vi "Top Level FPGA_w8randLED.vi"() -> ()   [LabVIEW 2012]
uses:
  <vilib>/Platform/TimedLoop/XDataNode/timing_clust.ctl
  <vilib>/Platform/TimedLoop/XDataNode/nitl_modes.ctl
  <vilib>/Platform/TimedLoop/XDataNode/wakeup.ctl
  <vilib>/rvi/DataTransferAndStorage/Container/Common/niFpgaContainerMetaDataKey.ctl
  <vilib>/rvi/DataTransferAndStorage/Container/Common/niFpgaContainerState.ctl
  <vilib>/rvi/DataTransferAndStorage/Container/Common/niFpgaDataTypeControl.ctl
  <vilib>/rvi/DataTransferAndStorage/Container/Common/niFpgaContainerImplementationControl.ctl
  <vilib>/rvi/DataTransferAndStorage/Container/Common/niFpgaContainerArbitrationOptionsControl.ctl
  <vilib>/rvi/DataTransferAndStorage/Container/Common/niFpgaTransferTypeControl.ctl
  <vilib>/rvi/DataTransferAndStorage/Container/Common/niFpgaContainerInitializationParameters.ctl
  <vilib>/rvi/Memory/Memory_Types/niFpgaMemoryInterfaceConfiguration.ctl
  <vilib>/rvi/FIFO/Fifo_Types/niFpgaFifoControlLogicControl.ctl
  <vilib>/rvi/eio/common/nirviEmuTemplateMethod_errors.vi
  <vilib>/rvi/FIFO/Fifo_Resource/nirvififoEmulationSetSize.vi
  <vilib>/rvi/DataTransferAndStorage/Container/Common/niFpgaContainerGetUniqueNameForEmu.vi
  <vilib>/rvi/Emulation/niFpgaSctlEmulationRegisterWithScheduler.vi
  <vilib>/rvi/DataTransferAndStorage/Container/Common/niFpgaContainerSetEmuInfo.vi
  <vilib>/rvi/eio/common/nirviEmuReportErrorAndStop.vi
  <vilib>/rvi/Emulation/niFpgaSctlEmulationScheduler.vi
  <vilib>/rvi/Emulation/niFpgaSctlEmulationFifoFullMgr.vi
  <vilib>/rvi/errors/niFpgaSetErrorForExecOnDevCompSimple.vi
  <vilib>/rvi/Memory/Memory_Emulation/nirvimemoryEmulationManagerCache_GetValue.vi
  <vilib>/rvi/Memory/Memory_Emulation/niFpgaMemoryEmulationValidateCache.vi
  <vilib>/rvi/Memory/Memory_Emulation/nirvimemoryEmulationManagerCache_InsertValue.vi
  <vilib>/rvi/Memory/Memory_Emulation/nirvimemoryEmulationManagerCache_SetValue.vi
  <vilib>/rvi/Emulation/niFpgaSctlEmulationResourceMgr.vi
  <vilib>/rvi/Memory/Memory_Emulation/niFpgaMemoryEmulationCacheClearOnFirstRun.vi
  <vilib>/rvi/Memory/Memory_Emulation/nirvimemoryEmulationManagerCache_MakeExclusive.vi
  <vilib>/rvi/Memory/Memory_Emulation/nirvimemoryEmulationManagerCache_ReleaseExclusive.vi
  <vilib>/Utility/error.llb/Clear Errors.vi
  <vilib>/eio/EIONode/EIONode.xnode
  <vilib>/rvi/DataTransferAndStorage/Container/XNode/niFpgaContainer.xnode
  <vilib>/rvi/FIFO/Fifo_Resource/nirvififoEmulationClear.vi
  <vilib>/Platform/TimedLoop/XDataNode/XDataNode.xnode
  <vilib>/rvi/LocalResourceManager/LocalResourceManager.xnode
  <vilib>/rvi/FIFO/Fifo_Resource/nirvififoEmulationRead.vi
  <vilib>/rvi/DataTransferAndStorage/Register/Emulation/niFpgaRegisterEmulation.vi
  <vilib>/rvi/Memory/Memory_Emulation/nirvimemoryEmulation.vi
  <vilib>/rvi/FIFO/Fifo_Resource/nirvififoEmulationWrite.vi
  <vilib>/Platform/TimedLoop/XDataNode/XDNodeRunTimeDep.lvlib
panel:
  out "Total number of pulses sent":u64
  in  "location":i16(ring) items=["Purdue", "NIKHEF", "Zurich", "???"]
  in  "Testpulse duration (20 ns ticks)":u32
  in  "initial value":u64
  in  "channel 7 on/off":bool
  in  "channel 6 on/off":bool
  in  "channel 5 on/off":bool
  in  "channel 4 on/off":bool
  in  "channel 3 on/off":bool
  in  "channel 1 on/off":bool
  in  "channel 2 on/off":bool
  in  "channel 0 on/off":bool
  out "Timestamp":u64
  in  "Stop FPGA and exit":bool
  out "DMA FIFO Timed Out?":bool
  in  "Testpulser On/Off":bool
  in  "Testpulse Time Delay (20 ns ticks)":u32=15
  in  "circular buffer length":u32=1000
  in  "# of pretrigger":u32=20
  out "IO Module\\Pll Unlocked":bool
  out "IO Module\\ADC Error B":bool
  out "IO Module\\ADC Error A":bool
  out "Init Done":bool
  in  "Trigger 4":i16=4000
  in  "Trigger 5":i16=4000
  in  "Trigger 6":i16=4000
  in  "Trigger 7":i16=4000
  in  "Trigger 2":i16=4000
  in  "Trigger 3":i16=4000
  in  "Trigger 1":i16=4000
  in  "Record Size only data":u32=95
  in  "Trigger 0":i16=4000
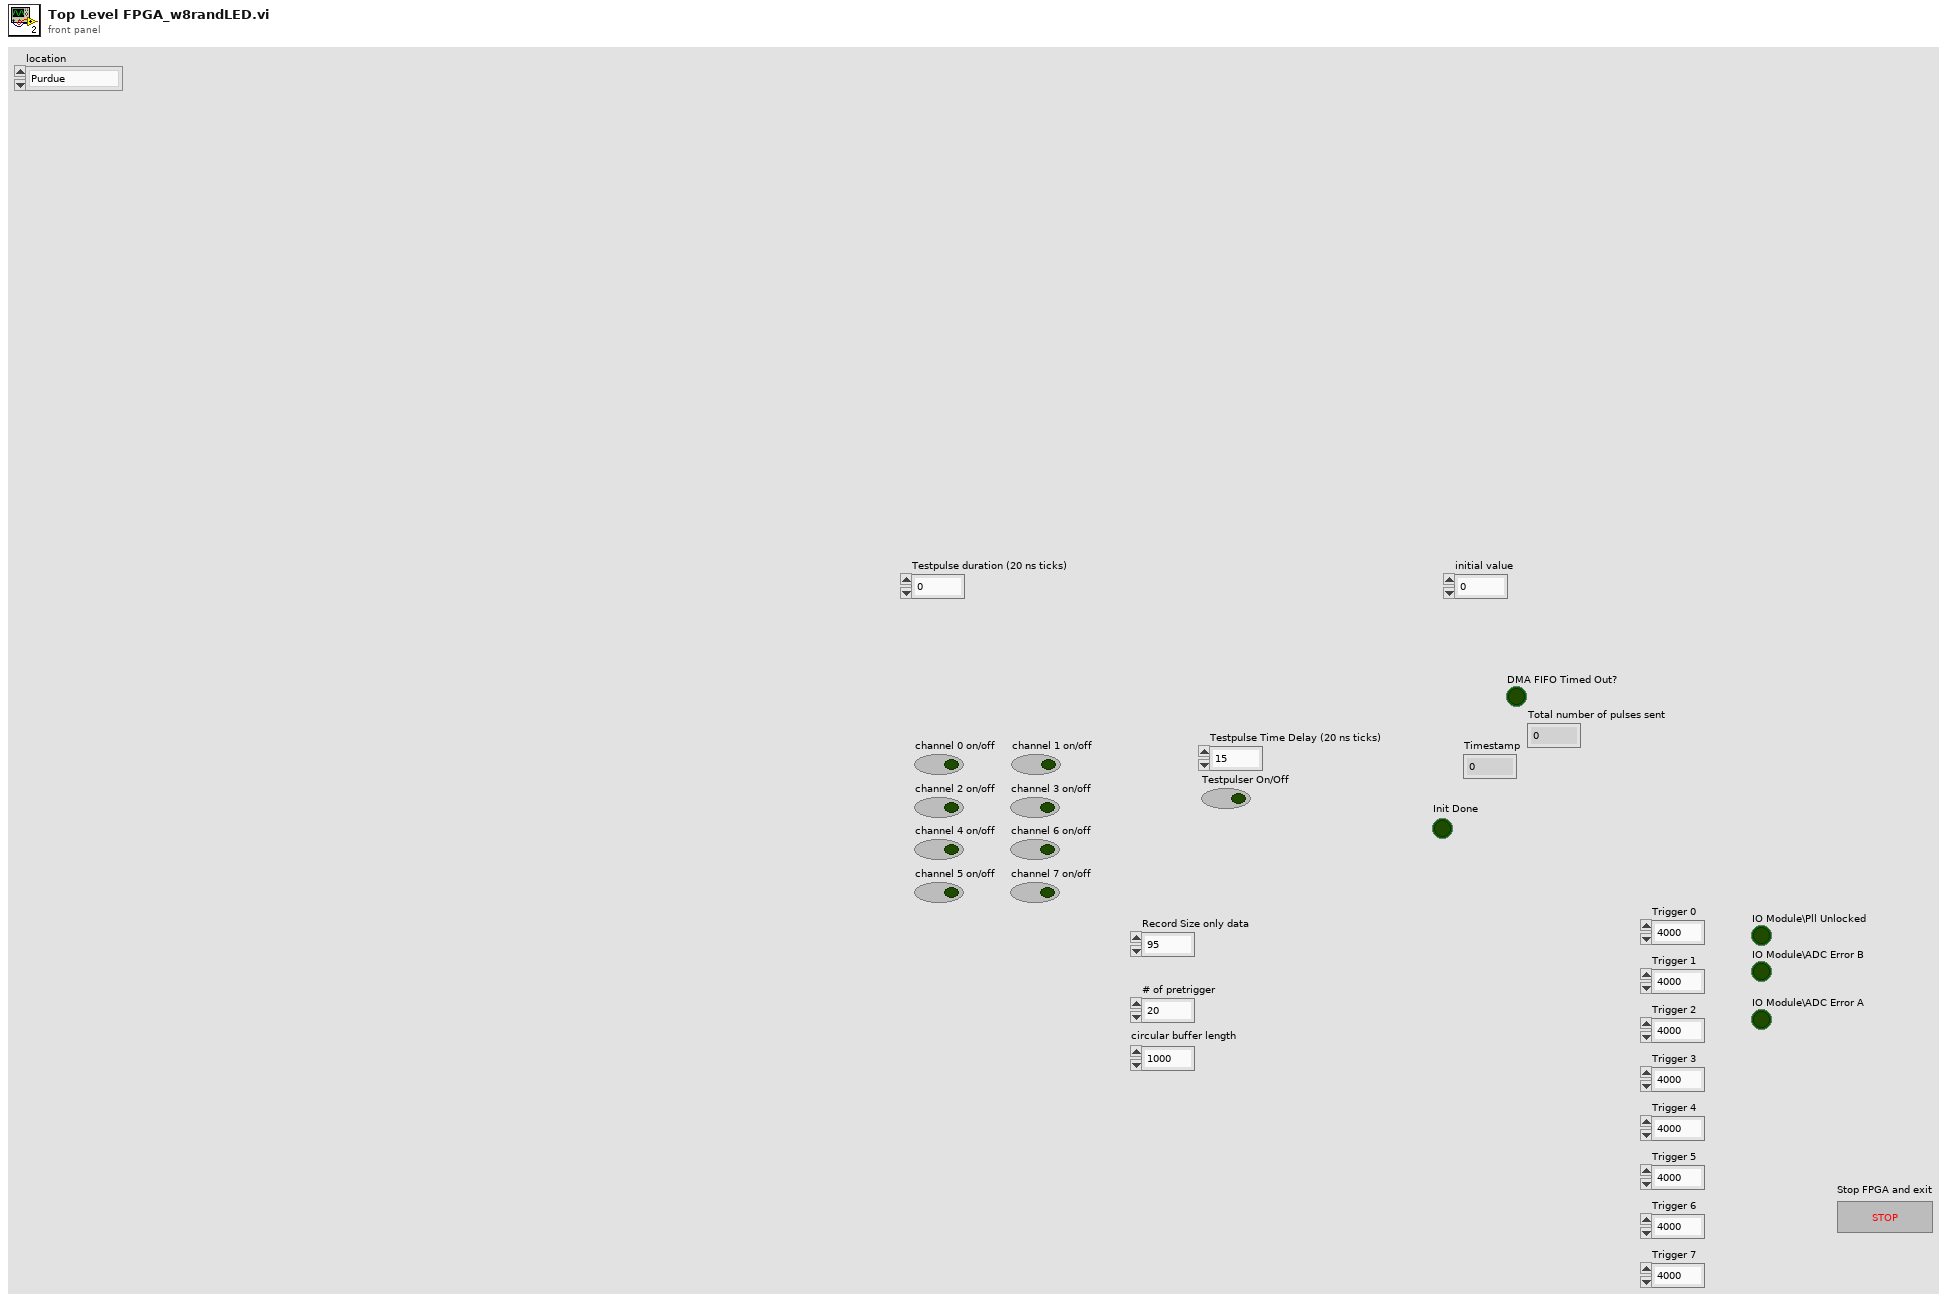
[diagram p1: front panel]
types:
  T1 = typedef "XDNodeRunTimeDep.lvlib/timing_clust.ctl" = cluster{"Expected End [f-1]":u64, "Actual End [f-1]":u64, "Finished Late? [f-1]":bool, "Expected End [i-1]":u64, "Actual End [i-1]":u64, "Finished Late? [i-1]":bool, "Expected Start [i]":u64, "Actual Start [i]":u64, "Expected Start [f]":u64, "Actual Start [f]":u64, "Source Name":string, "Structure Name":string, "Period":i64, "Deadline":i64, "Offset":i64, "Start":i64, "Priority":i32, "Timeout":i32, "Mode":T2, "Wakeup Reason":T3, "Error":errorcluster, "Source Type":string, "Secondary Source Type":string, "Global End Time":u64, "Global Start Time":u64, "Frame Duration":u64, "Iteration Duration":u64, "Assigned CPU":i32, "I/O Scan Engine Mode":u32}
  T2 = typedef "XDNodeRunTimeDep.lvlib/nitl_modes.ctl" = enum32{"No Change", "Process missed periods, maintain original phase", "Discard missed periods, maintain original phase", "Process missed periods, ignore original phase", "Discard missed periods, ignore original phase"}
  T3 = typedef "XDNodeRunTimeDep.lvlib/wakeup.ctl" = enum32{"Normal", "Aborted", "Asynchronous wakeup", "Timing source error", "Timed loop error", "Timeout"}
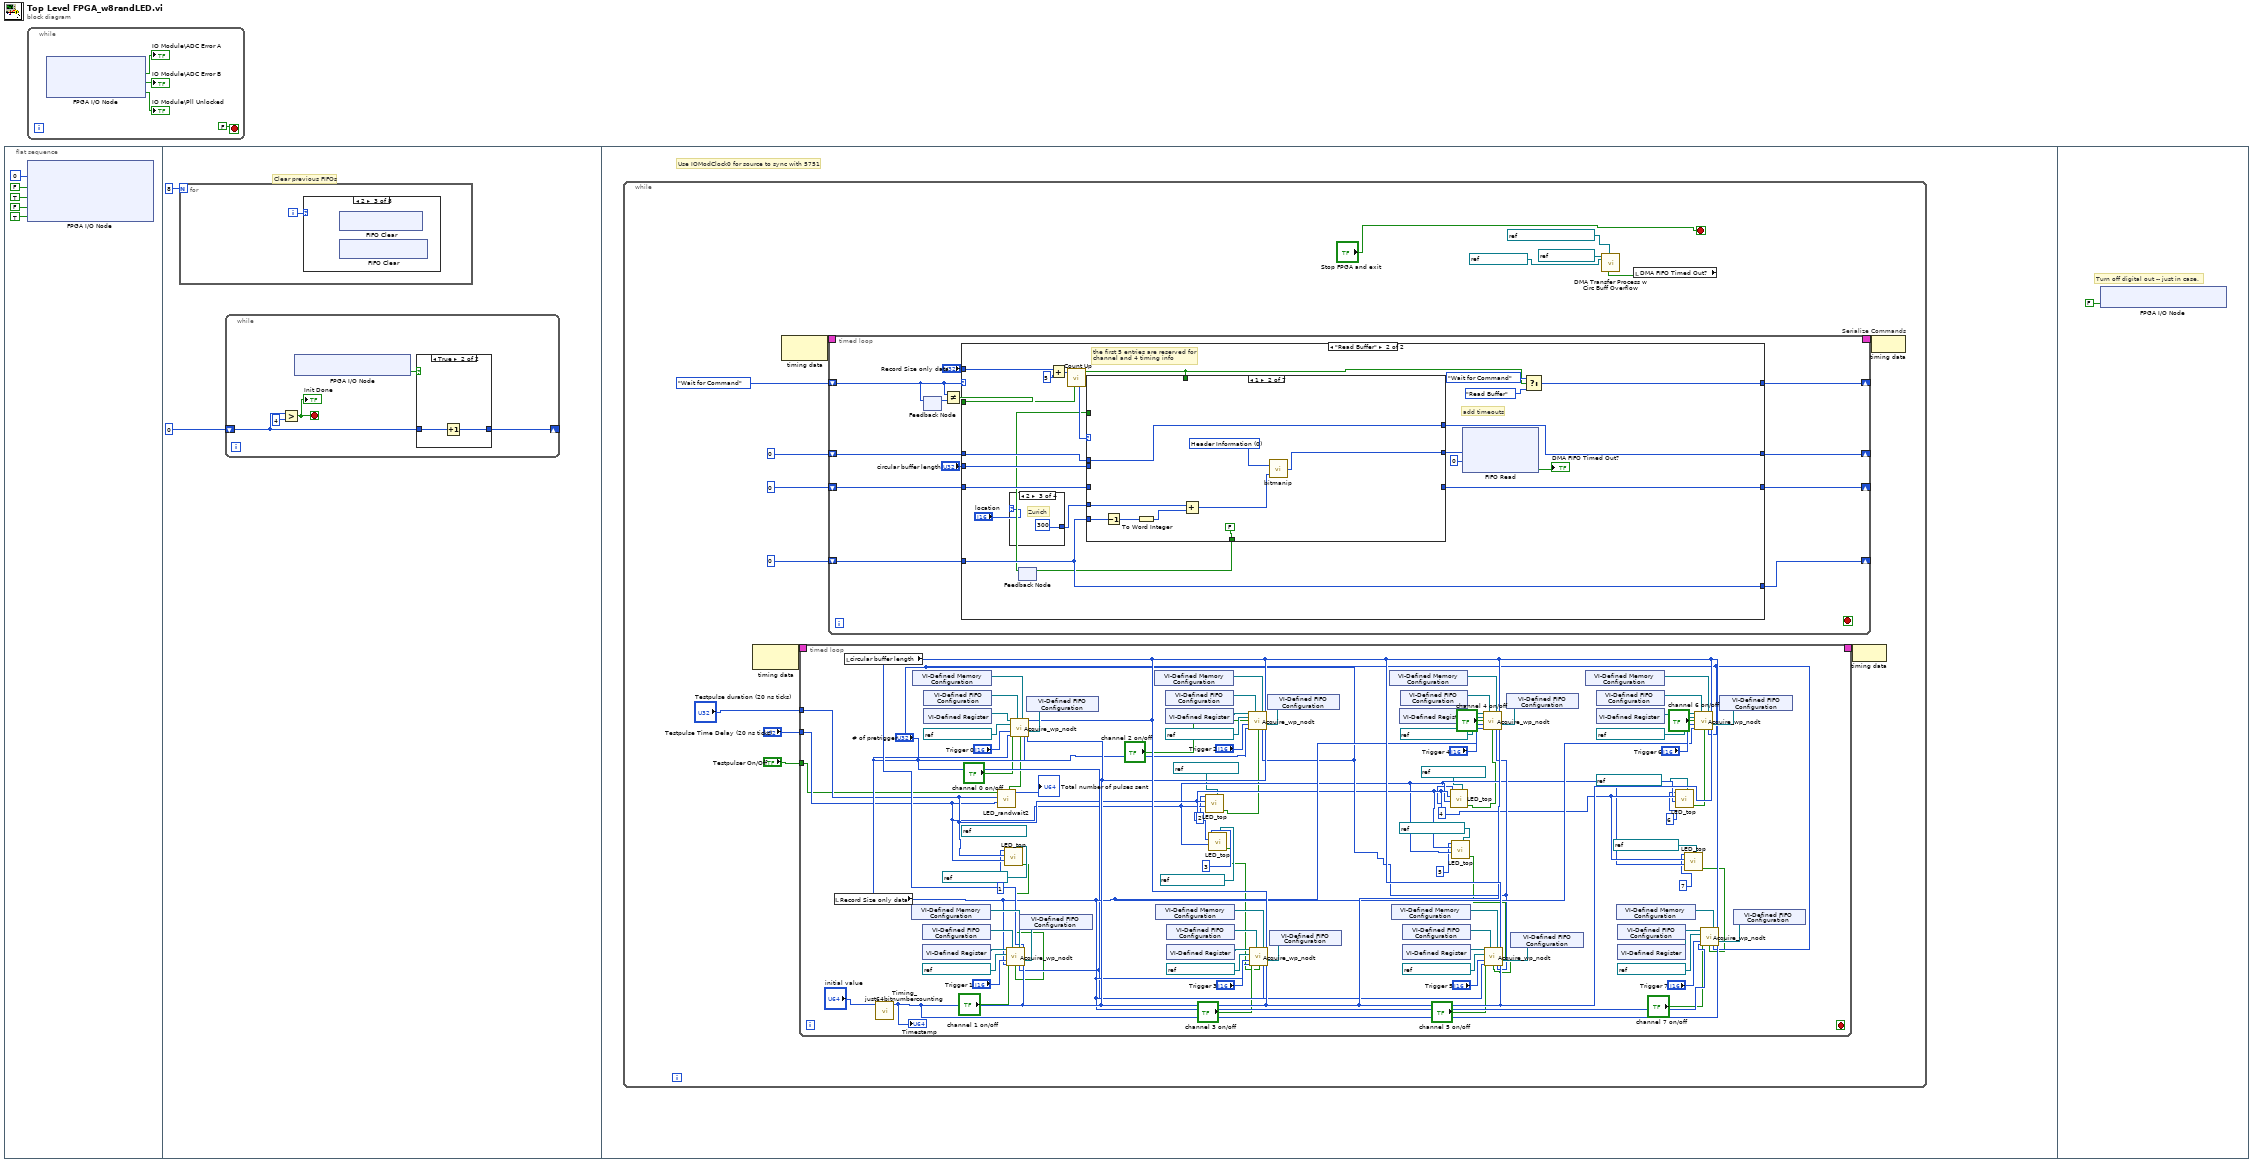
[diagram p0: block diagram]
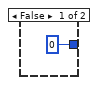
[diagram p2: hidden frame]
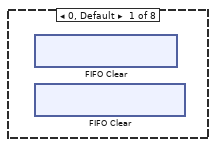
[diagram p3: hidden frame]
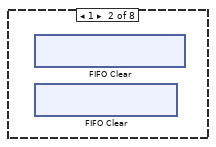
[diagram p4: hidden frame]
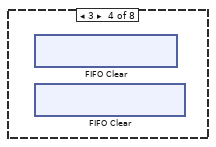
[diagram p5: hidden frame]
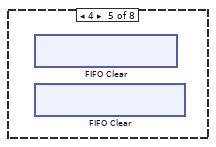
[diagram p6: hidden frame]
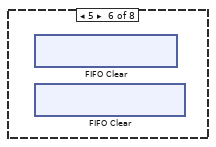
[diagram p7: hidden frame]
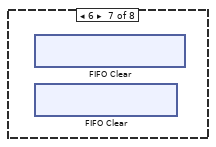
[diagram p8: hidden frame]
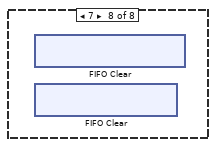
[diagram p9: hidden frame]
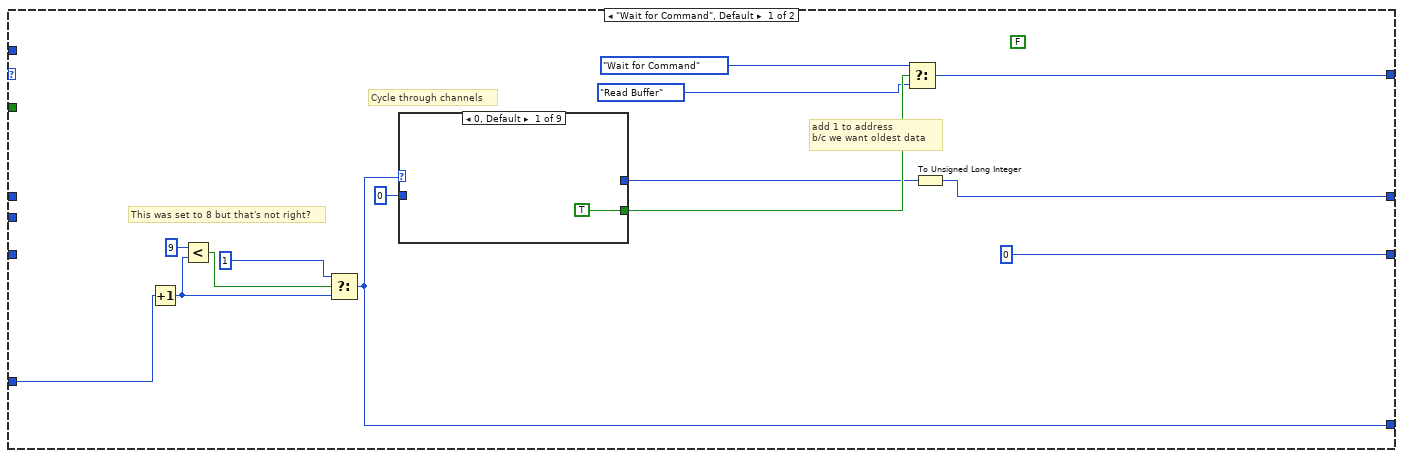
[diagram p10: hidden frame]
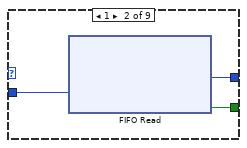
[diagram p11: hidden frame]
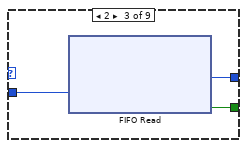
[diagram p12: hidden frame]
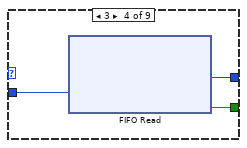
[diagram p13: hidden frame]
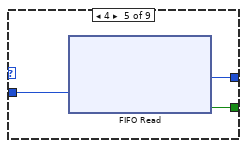
[diagram p14: hidden frame]
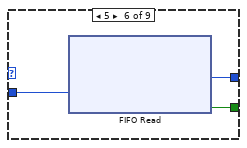
[diagram p15: hidden frame]
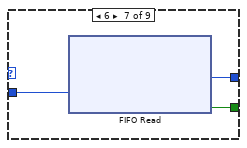
[diagram p16: hidden frame]
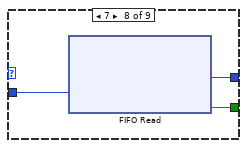
[diagram p17: hidden frame]
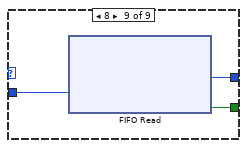
[diagram p18: hidden frame]
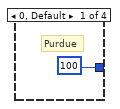
[diagram p19: hidden frame]
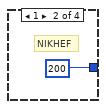
[diagram p20: hidden frame]
diagram:
  n1 = flat-sequence {
    frame #0 {
      n2 = xnode "FPGA I/O Node"("IO Module\\Sample Clock Select"=u8 0 ("IO Module\\Sample Clock Select"), "IO Module\\Force Initialization"=FALSE ("IO Module\\Force Initialization"), "IO Module\\Force Initialization"=TRUE ("IO Module\\Force Initialization"), "IO Module\\Force Initialization"=FALSE ("IO Module\\Force Initialization"), "IO Module\\Digital Output Enable"=TRUE ("IO Module\\Digital Output Enable")) -> ()  [unwired: 5 in, 5 out]
    }
    frame #1 {
      # "Clear previous FIFOs"
      n3 = for {
        N: 8 -> [_]
        i -> [w16]
        n4 = case shown="2" w16 {
          frame 0, Default {
            n5 = xnode ("FIFO Clear")() -> ()  [unwired: 1 in, 1 out]
            n6 = xnode ("FIFO Clear")() -> ()  [unwired: 1 in, 1 out]
          }
          frame 1 {
            n7 = xnode ("FIFO Clear")() -> ()  [unwired: 1 in, 1 out]
            n8 = xnode ("FIFO Clear")() -> ()  [unwired: 1 in, 1 out]
          }
          frame 2 {
            n9 = xnode ("FIFO Clear")() -> ()  [unwired: 1 in, 1 out]
            n10 = xnode ("FIFO Clear")() -> ()  [unwired: 1 in, 1 out]
          }
          frame 3 {
            n11 = xnode ("FIFO Clear")() -> ()  [unwired: 1 in, 1 out]
            n12 = xnode ("FIFO Clear")() -> ()  [unwired: 1 in, 1 out]
          }
          frame 4 {
            n13 = xnode ("FIFO Clear")() -> ()  [unwired: 1 in, 1 out]
            n14 = xnode ("FIFO Clear")() -> ()  [unwired: 1 in, 1 out]
          }
          frame 5 {
            n15 = xnode ("FIFO Clear")() -> ()  [unwired: 1 in, 1 out]
            n16 = xnode ("FIFO Clear")() -> ()  [unwired: 1 in, 1 out]
          }
          frame 6 {
            n17 = xnode ("FIFO Clear")() -> ()  [unwired: 1 in, 1 out]
            n18 = xnode ("FIFO Clear")() -> ()  [unwired: 1 in, 1 out]
          }
          frame 7 {
            n19 = xnode ("FIFO Clear")() -> ()  [unwired: 1 in, 1 out]
            n20 = xnode ("FIFO Clear")() -> ()  [unwired: 1 in, 1 out]
          }
        }
      }
      n21 = while {
        shift-right: [w11] -> _
        shift-left: u16 0 -> [w10]
        stop <- w8 stop-if-true
        n22 = Greater?(x=w10, y=u16 4) -> (0:w8:bool)
        "Init Done" <- w8
        n23 = xnode "FPGA I/O Node"() -> ("IO Module\\Initialization Done"=w12:bool)  [unwired: 1 in, 1 out]
        n24 = case shown="True" w12 {
          tunnel: [u16 0 w15] -> w11
          tunnel: w10 -> [_ w14]
          frame False {
          }
          frame True {
            n25 = Increment(x=w14) -> (x+1=w15:u16)
          }
        }
      }
    }
    frame #2 {
      # "Use IOModClock0 for source to sync with 5751"
      n26 = while {
        stop <- "Stop FPGA and exit" stop-if-true
        n27 = node-c288() -> (w25:T1)  [unwired: 1 in]
        n28 = node-c288() -> (w27:T1)  [unwired: 1 in]
        n29 = timed-loop {
          timing: w25 -> [_]
          timing-out: [_] -> w24
          tunnel: "Testpulser On/Off" -> [w35]
          tunnel: "Testpulse Time Delay (20 ns ticks)" -> [w66]
          tunnel: "Testpulse duration (20 ns ticks)" -> [w67]
          stop <- _ stop-if-true
          (unwired) refnum<k21> "IO Module\\D0 0" ("FPGA I/O In")
          n30 = local read "Record Size only data"() -> (w70:u32)
          n31 = local read "circular buffer length"() -> (w72:u32)
          n32 = call "Timing_just64bitnumbercounting.vi"("initial value"="initial value") -> ("x+1"=w71:u64)  [unwired: 10 in]
          "Timestamp" <- w71
          n33 = xnode "VI-Defined Memory Configuration"() -> ("Memory Out"=w118:refnum<k21>)
          n34 = xnode "VI-Defined Memory Configuration"() -> ("Memory Out"=w73:refnum<k21>)
          n35 = xnode "VI-Defined FIFO Configuration"() -> ("FIFO Out"=w117:refnum<k21>)
          n36 = xnode "VI-Defined Register"() -> ("Register Out"=w98:refnum<k21>)
          n37 = xnode "VI-Defined FIFO Configuration"() -> ("FIFO Out"=w74:refnum<k21>)
          n38 = xnode "VI-Defined Register"() -> ("Register Out"=w69:refnum<k21>)
          n39 = call "LED_randwait2.vi"("Testpulse Time Delay (20 ns ticks)"=w66, "Testpulse duration (20 ns ticks)"=w67, "Testpulser On/Off"=w35) -> ("Total number of pulses sent"=→"Total number of pulses sent":u64, "Is Test Pulse?"=w34:bool)  [unwired: 7 in]
          n40 = call "LED_top.vi"("FPGA I/O In"=refnum<k21> "IO Module\\D0 1", "Testpulse Time Delay (20 ns ticks)"=w66, "Testpulse duration (20 ns ticks)"=w67, "Address In"=u16 1) -> ("Is Test Pulse?"=w36:bool)  [unwired: 6 in, 1 out]
          n41 = xnode "VI-Defined FIFO Configuration"() -> ("FIFO Out"=w84:refnum<k21>)
          n42 = call "Acquire_wp_nodt.vi"("Ch Armed Reg"=w98, "Command FIFO"=w117, "Circular Buffer Mem"=w118, "circular buffer length"=w72, "FPGA I/O In"=refnum<k21> "IO Module\\AI A1", "channel on/off"="channel 1 on/off", "Trigger"="Trigger 1", "Timing FIFO"=w84, "Samples to Acquire"=w70, "Is Test Pulse?"=w36, "# of pretrigger"="# of pretrigger", "timing"=w71) -> ()  [unwired: 4 in]
          n43 = xnode "VI-Defined FIFO Configuration"() -> ("FIFO Out"=w77:refnum<k21>)
          n44 = call "Acquire_wp_nodt.vi"("Ch Armed Reg"=w69, "Command FIFO"=w74, "Circular Buffer Mem"=w73, "circular buffer length"=w72, "FPGA I/O In"=refnum<k21> "IO Module\\AI A0", "channel on/off"="channel 0 on/off", "Trigger"="Trigger 0", "Timing FIFO"=w77, "Samples to Acquire"=w70, "Is Test Pulse?"=w34, "# of pretrigger"="# of pretrigger", "timing"=w71) -> ()  [unwired: 4 in]
          n45 = xnode "VI-Defined Memory Configuration"() -> ("Memory Out"=w112:refnum<k21>)
          n46 = xnode "VI-Defined Memory Configuration"() -> ("Memory Out"=w115:refnum<k21>)
          n47 = xnode "VI-Defined FIFO Configuration"() -> ("FIFO Out"=w111:refnum<k21>)
          n48 = xnode "VI-Defined Register"() -> ("Register Out"=w94:refnum<k21>)
          n49 = xnode "VI-Defined FIFO Configuration"() -> ("FIFO Out"=w116:refnum<k21>)
          n50 = xnode "VI-Defined Register"() -> ("Register Out"=w96:refnum<k21>)
          n51 = call "LED_top.vi"("FPGA I/O In"=refnum<k21> "IO Module\\D0 2", "Testpulse Time Delay (20 ns ticks)"=w66, "Testpulse duration (20 ns ticks)"=w67, "Address In"=u16 2 ("Total number of pulses sent")) -> ("Is Test Pulse?"=w42:bool)  [unwired: 6 in, 1 out]
          n52 = call "LED_top.vi"("FPGA I/O In"=refnum<k21> "IO Module\\D0 3", "Testpulse Time Delay (20 ns ticks)"=w66, "Testpulse duration (20 ns ticks)"=w67, "Address In"=u16 3 ("Total number of pulses sent")) -> ("Is Test Pulse?"=w37:bool)  [unwired: 6 in, 1 out]
          n53 = xnode "VI-Defined FIFO Configuration"() -> ("FIFO Out"=w83:refnum<k21>)
          n54 = call "Acquire_wp_nodt.vi"("Ch Armed Reg"=w94, "Command FIFO"=w111, "Circular Buffer Mem"=w112, "circular buffer length"=w72, "FPGA I/O In"=refnum<k21> "IO Module\\AI A2", "channel on/off"="channel 2 on/off", "Trigger"="Trigger 2", "Timing FIFO"=w83, "Samples to Acquire"=w70, "Is Test Pulse?"=w42, "# of pretrigger"="# of pretrigger", "timing"=w71) -> ()  [unwired: 4 in]
          n55 = xnode "VI-Defined FIFO Configuration"() -> ("FIFO Out"=w82:refnum<k21>)
          n56 = call "Acquire_wp_nodt.vi"("Ch Armed Reg"=w96, "Command FIFO"=w116, "Circular Buffer Mem"=w115, "circular buffer length"=w72, "FPGA I/O In"=refnum<k21> "IO Module\\AI A3", "channel on/off"="channel 3 on/off", "Trigger"="Trigger 3", "Timing FIFO"=w82, "Samples to Acquire"=w70, "Is Test Pulse?"=w37, "# of pretrigger"="# of pretrigger", "timing"=w71) -> ()  [unwired: 4 in]
          n57 = xnode "VI-Defined Memory Configuration"() -> ("Memory Out"=w100:refnum<k21>)
          n58 = xnode "VI-Defined Memory Configuration"() -> ("Memory Out"=w103:refnum<k21>)
          n59 = xnode "VI-Defined Register"() -> ("Register Out"=w88:refnum<k21>)
          n60 = xnode "VI-Defined FIFO Configuration"() -> ("FIFO Out"=w99:refnum<k21>)
          n61 = xnode "VI-Defined FIFO Configuration"() -> ("FIFO Out"=w104:refnum<k21>)
          n62 = xnode "VI-Defined Register"() -> ("Register Out"=w92:refnum<k21>)
          n63 = call "LED_top.vi"("FPGA I/O In"=refnum<k21> "IO Module\\D0 4", "Testpulse Time Delay (20 ns ticks)"=w66, "Testpulse duration (20 ns ticks)"=w67, "Address In"=u16 4 ("Total number of pulses sent")) -> ("Is Test Pulse?"=w41:bool)  [unwired: 6 in, 1 out]
          n64 = call "LED_top.vi"("FPGA I/O In"=refnum<k21> "IO Module\\D0 5", "Testpulse Time Delay (20 ns ticks)"=w66, "Testpulse duration (20 ns ticks)"=w67, "Address In"=u16 5 ("Total number of pulses sent")) -> ("Is Test Pulse?"=w38:bool)  [unwired: 6 in, 1 out]
          n65 = xnode "VI-Defined FIFO Configuration"() -> ("FIFO Out"=w81:refnum<k21>)
          n66 = call "Acquire_wp_nodt.vi"("Ch Armed Reg"=w88, "Command FIFO"=w99, "Circular Buffer Mem"=w100, "circular buffer length"=w72, "FPGA I/O In"=refnum<k21> "IO Module\\AI A4", "channel on/off"="channel 4 on/off", "Trigger"="Trigger 4", "Timing FIFO"=w81, "Samples to Acquire"=w70, "Is Test Pulse?"=w41, "# of pretrigger"="# of pretrigger", "timing"=w71) -> ()  [unwired: 4 in]
          n67 = xnode "VI-Defined FIFO Configuration"() -> ("FIFO Out"=w80:refnum<k21>)
          n68 = call "Acquire_wp_nodt.vi"("Ch Armed Reg"=w92, "Command FIFO"=w104, "Circular Buffer Mem"=w103, "circular buffer length"=w72, "FPGA I/O In"=refnum<k21> "IO Module\\AI A5", "channel on/off"="channel 5 on/off", "Trigger"="Trigger 5", "Timing FIFO"=w80, "Samples to Acquire"=w70, "Is Test Pulse?"=w38, "# of pretrigger"="# of pretrigger", "timing"=w71) -> ()  [unwired: 4 in]
          n69 = xnode "VI-Defined Memory Configuration"() -> ("Memory Out"=w109:refnum<k21>)
          n70 = xnode "VI-Defined FIFO Configuration"() -> ("FIFO Out"=w110:refnum<k21>)
          n71 = xnode "VI-Defined Register"() -> ("Register Out"=w90:refnum<k21>)
          n72 = xnode "VI-Defined Memory Configuration"() -> ("Memory Out"=w106:refnum<k21>)
          n73 = xnode "VI-Defined FIFO Configuration"() -> ("FIFO Out"=w105:refnum<k21>)
          n74 = xnode "VI-Defined Register"() -> ("Register Out"=w86:refnum<k21>)
          n75 = call "LED_top.vi"("FPGA I/O In"=refnum<k21> "IO Module\\D0 6", "Testpulse Time Delay (20 ns ticks)"=w66, "Testpulse duration (20 ns ticks)"=w67, "Address In"=u16 6 ("Total number of pulses sent")) -> ("Is Test Pulse?"=w40:bool)  [unwired: 6 in, 1 out]
          n76 = call "LED_top.vi"("FPGA I/O In"=refnum<k21> "IO Module\\D0 7", "Testpulse Time Delay (20 ns ticks)"=w66, "Testpulse duration (20 ns ticks)"=w67, "Address In"=u16 7 ("Total number of pulses sent")) -> ("Is Test Pulse?"=w39:bool)  [unwired: 6 in, 1 out]
          n77 = xnode "VI-Defined FIFO Configuration"() -> ("FIFO Out"=w79:refnum<k21>)
          n78 = call "Acquire_wp_nodt.vi"("Ch Armed Reg"=w90, "Command FIFO"=w110, "Circular Buffer Mem"=w109, "circular buffer length"=w72, "FPGA I/O In"=refnum<k21> "IO Module\\AI A6", "channel on/off"="channel 6 on/off", "Trigger"="Trigger 6", "Timing FIFO"=w79, "Samples to Acquire"=w70, "Is Test Pulse?"=w40, "# of pretrigger"="# of pretrigger", "timing"=w71) -> ()  [unwired: 4 in]
          n79 = xnode "VI-Defined FIFO Configuration"() -> ("FIFO Out"=w78:refnum<k21>)
          n80 = call "Acquire_wp_nodt.vi"("Ch Armed Reg"=w86, "Command FIFO"=w105, "Circular Buffer Mem"=w106, "circular buffer length"=w72, "FPGA I/O In"=refnum<k21> "IO Module\\AI A7", "channel on/off"="channel 7 on/off", "Trigger"="Trigger 7", "Timing FIFO"=w78, "Samples to Acquire"=w70, "Is Test Pulse?"=w39, "# of pretrigger"="# of pretrigger", "timing"=w71) -> ()  [unwired: 4 in]
        }
        n81 = timed-loop "Serialize Commands" {
          timing: w27 -> [_]
          timing-out: [_] -> w26
          shift-right: [w898] -> _
          shift-left: enum16{"Wait for Command", "Read Buffer"}."Wait for Command" -> [w896]
          shift-right: [w902] -> _
          shift-left: u32 0 ("Element") -> [w901]
          shift-right: [w900] -> _
          shift-left: u8 0 ("t") -> [w899]
          shift-right: [w893] -> _
          shift-left: u64 0 ("Element") -> [w892]
          stop <- _ stop-if-true
          n82 = feedback-in #1(w896) -> ()
          n83 = feedback #1() -> (w897:enum16{"Wait for Command", "Read Buffer"})  [unwired: 1 in]
          n84 = Not Equal?(x=w896, y=w897) -> (x != y?=w894:bool)
          n85 = case shown="\"Read Buffer\"" w896 {
            tunnel: "Record Size only data" -> [_ w953]
            tunnel: [w906 w963] -> w900
            tunnel: w899 -> [w908 w963]
            tunnel: [w909 w948] -> w902
            tunnel: w901 -> [_ w962]
            tunnel: [w912 w964] -> w898
            tunnel: "circular buffer length" -> [_ w961]
            tunnel: w894 -> [_ w955]
            tunnel: [u64 0 ("Element") w950] -> w893
            tunnel: w892 -> [_ w949]
            frame "Wait for Command", Default {
              (unwired) FALSE
              # "This was set to 8 but that's not right?"
              # "add 1 to address\nb/c we want oldest data"
              # "Cycle through channels"
              n86 = Increment(x=w908) -> (x+1=w907:u8)
              n87 = Less?(x=u8 9, y=w907) -> (x < y?=w916:bool)
              n88 = Select(t=u8 1, s=w916, f=w907) -> (s? t:f=w906:u8)
              n89 = case shown="0, Default" w906 {
                tunnel: [TRUE ("Timed Out?") w921 w922 w925 w928 w931 w934 w937 w940] -> w913
                tunnel: 0 ("Timeout") -> [_ w920 w924 w927 w930 w933 w936 w939 w942]
                tunnel: [_ w919 w923 w926 w929 w932 w935 w938 w941] -> w905
                frame 0, Default {
                }
                frame 1 {
                  n90 = xnode ("FIFO Read")("Timeout"=w920) -> ("Element"=w919:i16, "Timed Out?"=w921:bool)  [unwired: 1 in, 1 out]
                }
                frame 2 {
                  n91 = xnode ("FIFO Read")("Timeout"=w924) -> ("Element"=w923:i16, "Timed Out?"=w922:bool)  [unwired: 1 in, 1 out]
                }
                frame 3 {
                  n92 = xnode ("FIFO Read")("Timeout"=w927) -> ("Element"=w926:i16, "Timed Out?"=w925:bool)  [unwired: 1 in, 1 out]
                }
                frame 4 {
                  n93 = xnode ("FIFO Read")("Timeout"=w930) -> ("Element"=w929:i16, "Timed Out?"=w928:bool)  [unwired: 1 in, 1 out]
                }
                frame 5 {
                  n94 = xnode ("FIFO Read")("Timeout"=w933) -> ("Element"=w932:i16, "Timed Out?"=w931:bool)  [unwired: 1 in, 1 out]
                }
                frame 6 {
                  n95 = xnode ("FIFO Read")("Timeout"=w936) -> ("Element"=w935:i16, "Timed Out?"=w934:bool)  [unwired: 1 in, 1 out]
                }
                frame 7 {
                  n96 = xnode ("FIFO Read")("Timeout"=w939) -> ("Element"=w938:i16, "Timed Out?"=w937:bool)  [unwired: 1 in, 1 out]
                }
                frame 8 {
                  n97 = xnode ("FIFO Read")("Timeout"=w942) -> ("Element"=w941:i16, "Timed Out?"=w940:bool)  [unwired: 1 in, 1 out]
                }
              }
              n98 = Select(t=enum16{"Wait for Command", "Read Buffer"}."Wait for Command", s=w913, f=enum16{"Wait for Command", "Read Buffer"}."Read Buffer") -> (s? t:f=w912:enum16{"Wait for Command", "Read Buffer"})
              n99 = To Unsigned Long Integer(number=w905) -> (unsigned 32bit integer=w909:u32)
            }
            frame "Read Buffer" {
              # "the first 5 entries are reserved for channel and 4 timing info"
              # "add timeouts"
              n100 = case shown="2" "location" {
                tunnel: [i16 100 i16 200 i16 300 i16 400] -> w943
                frame 0, Default {
                  # "Purdue"
                }
                frame 1 {
                  # "NIKHEF"
                }
                frame 2 {
                  # "Zurich"
                }
                frame 3 {
                  # "???"
                }
              }
              n101 = feedback #2() -> (w947:bool)  [unwired: 1 in]
              n102 = Add(x=w953, y=u32 5) -> (x+y=w951:u32)
              n103 = call "Count Up.vi"("Reset?"=w955, "goal"=w951) -> ("Count Met"=w957:bool, "count"=w954:u32)  [unwired: 8 in]
              n104 = case shown="1" w954 {
                tunnel: w963 -> [_ w976 w984 _ _ _ w1023]
                tunnel: w962 -> [_ w981 w986 w1007 w1013 w1019 w1030]
                tunnel: w961 -> [_ _ _ _ _ _ w1029]
                tunnel: w957 -> [_ _ _ _ _ _ w1028]
                tunnel: [i16 0 ("Data") w979 w988 w1005 w1011 w1017 w1024] -> w956
                tunnel: w947 -> [_ _ _ _ _ _ w1026]
                tunnel: [u64 0 ("Element") _ w985 w1008 w1014 w1020 _] -> w950
                tunnel: w949 -> [_ _ _ w1008 w1014 w1020 _]
                tunnel: [u32 0 ("Element") w981 w986 w1007 w1013 w1019 _] -> w948
                tunnel: [FALSE FALSE FALSE FALSE FALSE TRUE FALSE] -> w946
                tunnel: w943 -> [_ w974 _ _ _ _ _]
                frame 0, Default {
                }
                frame 1 {
                  w978 = u16 0 items=["Header Information", "Particle Pulse", "Test Pulse"] ("Pulse Type")
                  n105 = Decrement(x=w976) -> (x-1=w977:u8)
                  n106 = To Word Integer(number=w977) -> (16bit integer=w975:i16)
                  n107 = Add(x=w974, y=w975) -> (x+y=w973:i16)
                  n108 = call "bitmanip.vi"("Pulse Type"=w978, "Integer to be written"=w973) -> ("Integer Written"=w979:i16)  [unwired: 2 in]
                }
                frame 2 {
                  # "reads out the lsb of the timing information"
                  n109 = case shown="2" w984 {
                    tunnel: [_ w989 w991 w993 w995 w997 w999 w1001 w1003] -> w985
                    frame Default {
                    }
                    frame 1 {
                      n110 = xnode ("FIFO Read")("Timeout"=0) -> ("Element"=w989:u64)  [unwired: 1 in, 2 out]
                    }
                    frame 2 {
                      n111 = xnode ("FIFO Read")("Timeout"=0) -> ("Element"=w991:u64)  [unwired: 1 in, 2 out]
                    }
                    frame 3 {
                      n112 = xnode ("FIFO Read")("Timeout"=0) -> ("Element"=w993:u64)  [unwired: 1 in, 2 out]
                    }
                    frame 4 {
                      n113 = xnode ("FIFO Read")("Timeout"=0) -> ("Element"=w995:u64)  [unwired: 1 in, 2 out]
                    }
                    frame 5 {
                      n114 = xnode ("FIFO Read")("Timeout"=0) -> ("Element"=w997:u64)  [unwired: 1 in, 2 out]
                    }
                    frame 6 {
                      n115 = xnode ("FIFO Read")("Timeout"=0) -> ("Element"=w999:u64)  [unwired: 1 in, 2 out]
                    }
                    frame 7 {
                      n116 = xnode ("FIFO Read")("Timeout"=0) -> ("Element"=w1001:u64)  [unwired: 1 in, 2 out]
                    }
                    frame 8 {
                      n117 = xnode ("FIFO Read")("Timeout"=0) -> ("Element"=w1003:u64)  [unwired: 1 in, 2 out]
                    }
                  }
                  n118 = Split Number(x=w985) -> (hi(x)=w983:u32)  [unwired: 1 out]
                  n119 = Split Number(x=w983) -> (hi(x)=w982:u16)  [unwired: 1 out]
                  n120 = To Word Integer(number=w982) -> (16bit integer=w988:i16)
                }
                frame 3 {
                  n121 = Split Number(x=w1008) -> (hi(x)=w1010:u32)  [unwired: 1 out]
                  n122 = Split Number(x=w1010) -> (lo(x)=w1009:u16)  [unwired: 1 out]
                  n123 = To Word Integer(number=w1009) -> (16bit integer=w1005:i16)
                }
                frame 4 {
                  n124 = Split Number(x=w1014) -> (lo(x)=w1016:u32)  [unwired: 1 out]
                  n125 = Split Number(x=w1016) -> (hi(x)=w1015:u16)  [unwired: 1 out]
                  n126 = To Word Integer(number=w1015) -> (16bit integer=w1011:i16)
                }
                frame 5 {
                  n127 = Split Number(x=w1020) -> (lo(x)=w1022:u32)  [unwired: 1 out]
                  n128 = Split Number(x=w1022) -> (lo(x)=w1021:u16)  [unwired: 1 out]
                  n129 = To Word Integer(number=w1021) -> (16bit integer=w1017:i16)
                }
                frame 6.. {
                  n130 = call "Circular Buffer Address_try_without_deadtime.vi"("Reset?"=w1026, "Starting Address"=w1030, "circular buffer length"=w1029) -> ("Address"=w1027:u32)  [unwired: 8 in]
                  n131 = case shown="1" w1023 {
                    tunnel: w1027 -> [_ w1034 w1037 w1040 w1043 w1046 w1049 w1052 w1055]
                    tunnel: w1028 -> [_ w1033 w1036 w1039 w1042 w1045 w1048 w1051 w1054]
                    tunnel: [i16 0 w1032 w1035 w1038 w1041 w1044 w1047 w1050 w1053] -> w1024
                    frame Default {
                      # "Error"
                    }
                    frame 1 {
                      n132 = xnode ("Memory Read")("Address"=w1034) -> ("Data"=w1032:i16)  [unwired: 1 in, 1 out]
                      n133 = xnode ("Register Write")("Data"=w1033) -> ()  [unwired: 1 in, 1 out]
                    }
                    frame 2 {
                      n134 = xnode ("Memory Read")("Address"=w1037) -> ("Data"=w1035:i16)  [unwired: 1 in, 1 out]
                      n135 = xnode ("Register Write")("Data"=w1036) -> ()  [unwired: 1 in, 1 out]
                    }
                    frame 3 {
                      n136 = xnode ("Memory Read")("Address"=w1040) -> ("Data"=w1038:i16)  [unwired: 1 in, 1 out]
                      n137 = xnode ("Register Write")("Data"=w1039) -> ()  [unwired: 1 in, 1 out]
                    }
                    frame 4 {
                      n138 = xnode ("Memory Read")("Address"=w1043) -> ("Data"=w1041:i16)  [unwired: 1 in, 1 out]
                      n139 = xnode ("Register Write")("Data"=w1042) -> ()  [unwired: 1 in, 1 out]
                    }
                    frame 5 {
                      n140 = xnode ("Memory Read")("Address"=w1046) -> ("Data"=w1044:i16)  [unwired: 1 in, 1 out]
                      n141 = xnode ("Register Write")("Data"=w1045) -> ()  [unwired: 1 in, 1 out]
                    }
                    frame 6 {
                      n142 = xnode ("Memory Read")("Address"=w1049) -> ("Data"=w1047:i16)  [unwired: 1 in, 1 out]
                      n143 = xnode ("Register Write")("Data"=w1048) -> ()  [unwired: 1 in, 1 out]
                    }
                    frame 7 {
                      n144 = xnode ("Memory Read")("Address"=w1052) -> ("Data"=w1050:i16)  [unwired: 1 in, 1 out]
                      n145 = xnode ("Register Write")("Data"=w1051) -> ()  [unwired: 1 in, 1 out]
                    }
                    frame 8 {
                      n146 = xnode ("Memory Read")("Address"=w1055) -> ("Data"=w1053:i16)  [unwired: 1 in, 1 out]
                      n147 = xnode ("Register Write")("Data"=w1054) -> ()  [unwired: 1 in, 1 out]
                    }
                  }
                }
              }
              n148 = feedback-in #2(w946) -> ()
              n149 = xnode ("FIFO Read")("Element"=w956, "Timeout"=0) -> ("Timed Out?"=→"DMA FIFO Timed Out?":bool)  [unwired: 1 in, 1 out]
              n150 = Select(t=enum16{"Wait for Command", "Read Buffer"}."Wait for Command", s=w957, f=enum16{"Wait for Command", "Read Buffer"}."Read Buffer") -> (s? t:f=w964:enum16{"Wait for Command", "Read Buffer"})
            }
          }
        }
        n151 = local read "DMA FIFO Timed Out?"() -> (w30:bool)
        n152 = call "DMA Transfer Process w Circ Buff Overflow.vi"("DMA Write Timed Out?"=w30, "Clock Domain"=refnum<k21> "40 MHz Onboard Clock", "Local"=refnum<k21> "To DMA FIFO", "DMA"=refnum<k21> "To Host FIFO") -> ()  [unwired: 8 in]
        n153 = node-c288(w24) -> ()
        n154 = node-c288(w26) -> ()
      }
    }
    frame #3 {
      # "Turn off digital out -- just in case."
      n155 = xnode "FPGA I/O Node"("IO Module\\Digital Output Enable"=FALSE ("IO Module\\Digital Output Enable")) -> ()  [unwired: 1 in, 1 out]
    }
  }
  n156 = while {
    stop <- FALSE stop-if-true
    n157 = xnode "FPGA I/O Node"() -> ("IO Module\\ADC Error A"=→"IO Module\\ADC Error A":bool, "IO Module\\ADC Error B"=→"IO Module\\ADC Error B":bool, "IO Module\\Pll Unlocked"=→"IO Module\\Pll Unlocked":bool)  [unwired: 3 in, 3 out]
  }
